vi "AFG3022_Arb_Fun_Control.vi"(10 "Channel":u16(ring) items=["Channel 1", "Channel 2"], 11 "Function Selector":u16(ring)=3 items=["Sine", "Square", "Ramp", "Assymetric Sine", "Assymetric Arbitrary"]) -> ()   [LabVIEW 2011]
panel:
  in  "Set Zero Mean":bool
  out "Amplitude":dbl
  in  "Set Amplitude":bool
  out "Ts/T":dbl=0.32
  in  "Time Ratio":dbl[](array[slide])=[0.07, 0.15, 0.1, 0.6799999999999999] min=0.0 max=1.0 step=0.01 scale=0.0..1.0
  in  "Fine Amp":dbl(knob) min=0.0 max=1.0 step=0.1 scale=0.0..1.0
  in  "Course Amp":dbl(knob)=1.0 min=-10.0 max=10.0 step=1.0 scale=-10.0..10.0
  in  "Channel 2":bool
  in  "Channel 1":bool=TRUE
  in  "Set Frequency":bool
  in  "Scale":u16(ring)=2 items=["1", "10", "100", "1k", "10k"]
  in  "Fine Freq":dbl(knob)=0.30000000000000004 min=0.0 max=1.0 step=0.1 scale=0.0..1.0
  in  "Course Freq":dbl(knob)=3.0 min=0.0 max=10.0 step=1.0 scale=0.0..10.0
  in  "Stop Button":bool
  in  "VISA resource name":refnum<visa-resource-name>="USB0::0x0699::0x0347::C036837::INSTR"
  out "Frequency":dbl=330.0
  # "Suction Time"
  # "Blowing Time"
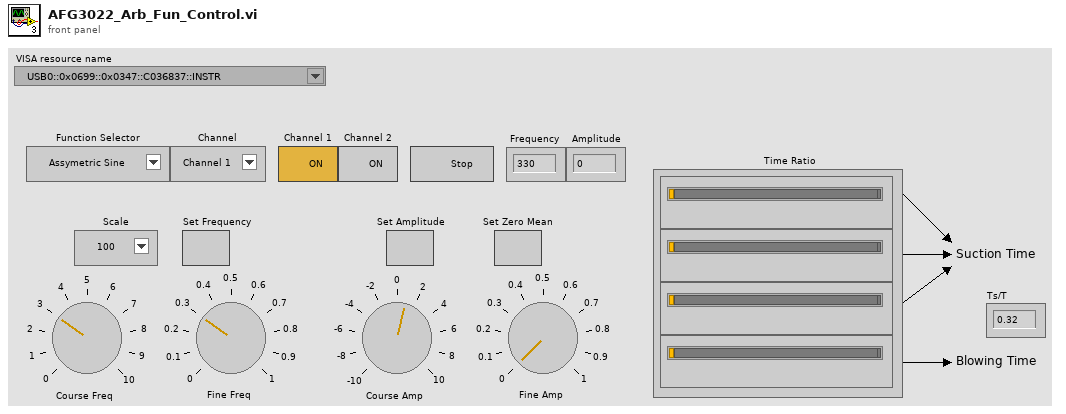
[diagram p1: front panel]
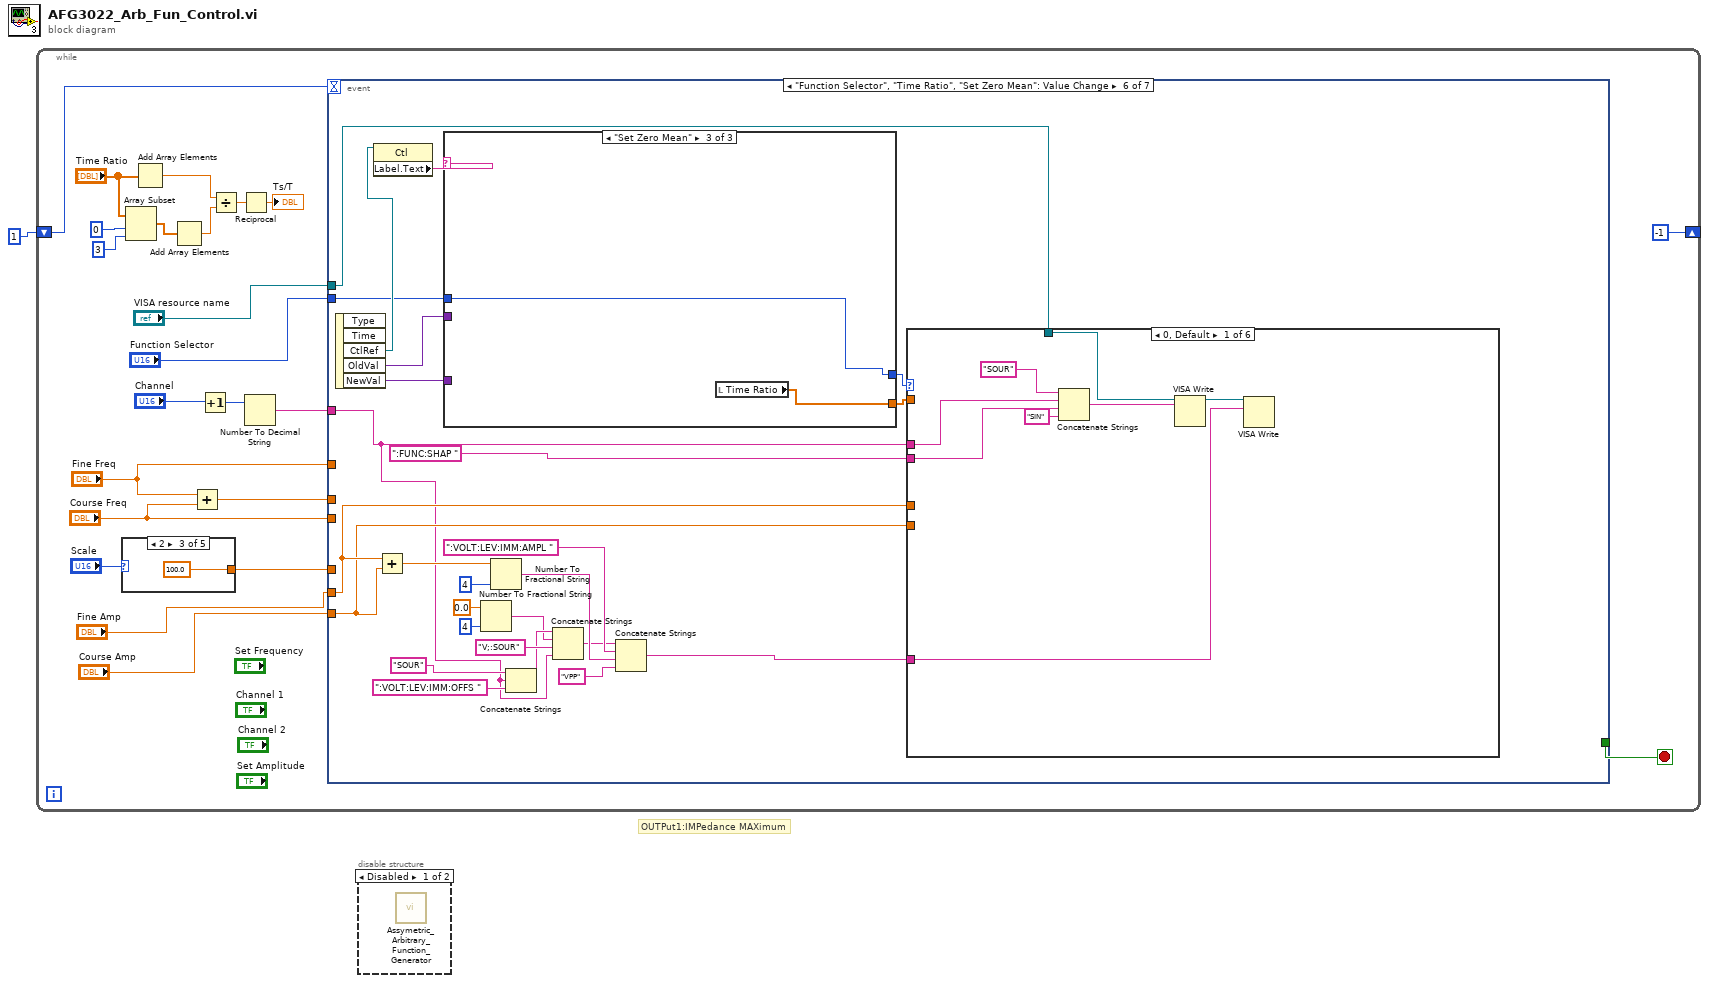
[diagram p0: block diagram]
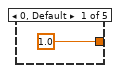
[diagram p3: hidden frame]
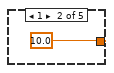
[diagram p4: hidden frame]
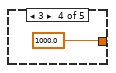
[diagram p5: hidden frame]
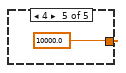
[diagram p6: hidden frame]
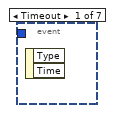
[diagram p7: hidden frame]
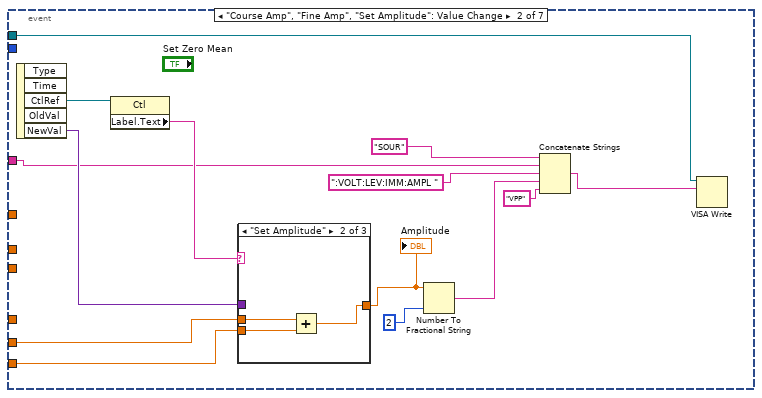
[diagram p8: hidden frame]
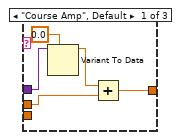
[diagram p9: hidden frame]
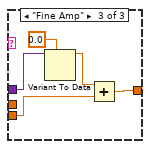
[diagram p10: hidden frame]
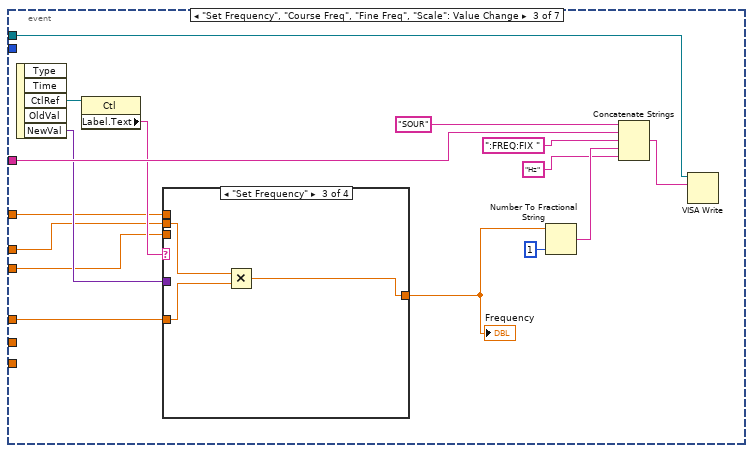
[diagram p11: hidden frame]
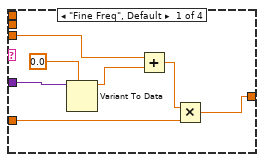
[diagram p12: hidden frame]
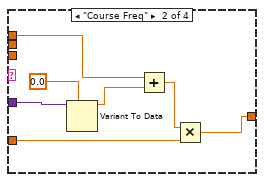
[diagram p13: hidden frame]
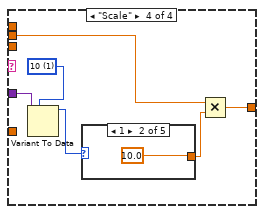
[diagram p14: hidden frame]
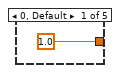
[diagram p15: hidden frame]
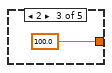
[diagram p16: hidden frame]
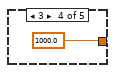
[diagram p17: hidden frame]
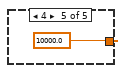
[diagram p18: hidden frame]
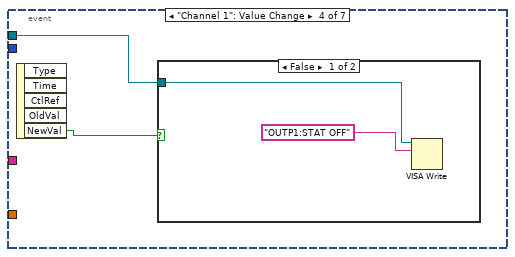
[diagram p19: hidden frame]
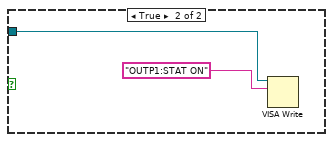
[diagram p20: hidden frame]
diagram:
  # "OUTPut1:IMPedance MAXimum"
  n1 = while {
    shift-right: [-1] -> _
    shift-left: 1 -> [w21]
    stop <- w23 stop-if-true
    n2 = case shown="2" "Scale" {
      tunnel: [1.0 10.0 100.0 1000.0 10000.0] -> w14
      frame 0, Default {
      }
      frame 1 {
      }
      frame 2 {
      }
      frame 3 {
      }
      frame 4 {
      }
    }
    n3 = Array Subset(array="Time Ratio", index=0, length=3) -> (w7:dbl[])
    n4 = Add Array Elements(numeric array="Time Ratio") -> (sum=w6:dbl)
    n5 = Add Array Elements(numeric array=w7) -> (sum=w5:dbl)
    n6 = Add(x="Fine Freq", y="Course Freq") -> (x+y=w16:dbl)
    n7 = Increment(x="Channel") -> (x+1=w19:u16)
    n8 = Divide(x=w6, y=w5) -> (x/y=w4:dbl)
    n9 = Reciprocal(x=w4) -> (1/x=→"Ts/T":dbl)
    n10 = Number To Decimal String(number=w19) -> (decimal integer string=w17:string)  [unwired: 1 in]
    n11 = event shown="[5] \"Function Selector\", \"Time Ratio\", \"Set Zero Mean\": Value Change" {
      selector: _ -> [_ _ _ _ _ _ _]
      dyn-events: _ -> [_ _ _ _ _ _ _]
      timeout: w21 -> [_ _ _ _ _ _ _]
      tunnel: "VISA resource name" -> [_ w30 w67 w102 w107 w138 _]
      tunnel: [_ _ _ _ _ _ "Stop Button"] -> w23
      tunnel: w17 -> [_ w31 w65 _ _ w116 _]
      tunnel: w16 -> [_ _ w61 _ _ _ _]
      tunnel: "Course Freq" -> [_ _ w59 _ _ _ _]
      tunnel: w14 -> [_ _ w58 _ _ _ _]
      tunnel: "Fine Freq" -> [_ _ w57 _ _ _ _]
      tunnel: "Course Amp" -> [_ w40 _ _ _ w118 _]
      tunnel: "Fine Amp" -> [_ w39 _ _ _ w119 _]
      tunnel: "Function Selector" -> [_ _ _ _ _ w114 _]
      event Timeout {
        n12 = event-data() -> ()  [unwired: 1 in, 2 out]
      }
      event "Course Amp", "Fine Amp", "Set Amplitude": Value Change {
        n13 = event-data() -> ("CtlRef"=w43:refnum<vi>, "NewVal"=w41:variant)  [unwired: 1 in, 3 out]
        n14 = property class="Ctl"(reference=w43) -> ("Label.Text"=w42:string)  [unwired: 1 in, 2 out]
        n15 = case shown="\"Set Amplitude\"" w42 {
          tunnel: w41 -> [w45 _ w53]
          tunnel: w40 -> [_ w50 w56]
          tunnel: w39 -> [w48 w51 _]
          tunnel: [w47 w49 w55] -> w38
          frame "Course Amp", Default {
            n16 = Variant To Data(type=0.0 ("Fine Amp"), Variant=w45) -> (data=w44:dbl)  [unwired: 1 in, 1 out]
            n17 = Add(x=w44, y=w48) -> (x+y=w47:dbl)
          }
          frame "Set Amplitude" {
            n18 = Add(x=w51, y=w50) -> (x+y=w49:dbl)
          }
          frame "Fine Amp" {
            n19 = Variant To Data(type=0.0 ("Fine Amp"), Variant=w53) -> (data=w52:dbl)  [unwired: 1 in, 1 out]
            n20 = Add(x=w52, y=w56) -> (x+y=w55:dbl)
          }
        }
        "Amplitude" <- w38
        n21 = Number To Fractional String(number=w38, precision (6)=i16 2) -> (F-format string=w33:string)  [unwired: 2 in]
        n22 = Concatenate Strings("SOUR" ("string"), w31, ":VOLT:LEV:IMM:AMPL " ("string"), w33, "VPP" ("string")) -> (w34:string)
        n23 = VISA Write(VISA resource name=w30, write buffer=w34) -> ()  [unwired: 1 in, 3 out]
      }
      event "Set Frequency", "Course Freq", "Fine Freq", "Scale": Value Change {
        n24 = event-data() -> ("CtlRef"=w64:refnum<vi>, "NewVal"=w62:variant)  [unwired: 1 in, 3 out]
        n25 = property class="Ctl"(reference=w64) -> ("Label.Text"=w63:string)  [unwired: 1 in, 2 out]
        n26 = case shown="\"Set Frequency\"" w63 {
          tunnel: w62 -> [w79 w86 _ w95]
          tunnel: w61 -> [_ _ w89 w91]
          tunnel: [w73 w80 w87 w90] -> w60
          tunnel: w59 -> [w76 _ _ _]
          tunnel: w58 -> [w74 w82 w88 _]
          tunnel: w57 -> [_ w81 _ _]
          frame "Fine Freq", Default {
            n27 = Variant To Data(type=0.0, Variant=w79) -> (data=w77:dbl)  [unwired: 1 in, 1 out]
            n28 = Add(x=w76, y=w77) -> (x+y=w75:dbl)
            n29 = Multiply(x=w75, y=w74) -> (x*y=w73:dbl)
          }
          frame "Course Freq" {
            n30 = Variant To Data(type=0.0, Variant=w86) -> (data=w84:dbl)  [unwired: 1 in, 1 out]
            n31 = Add(x=w81, y=w84) -> (x+y=w83:dbl)
            n32 = Multiply(x=w83, y=w82) -> (x*y=w80:dbl)
          }
          frame "Set Frequency" {
            n33 = Multiply(x=w89, y=w88) -> (x*y=w87:dbl)
          }
          frame "Scale" {
            w94 = u16 1 items=["1", "10", "100", "1k", "10k"] ("Scale")
            n34 = Variant To Data(type=w94, Variant=w95) -> (data=w93:u16)  [unwired: 1 in, 1 out]
            n35 = case shown="1" w93 {
              tunnel: [1.0 10.0 100.0 1000.0 10000.0] -> w92
              frame 0, Default {
              }
              frame 1 {
              }
              frame 2 {
              }
              frame 3 {
              }
              frame 4 {
              }
            }
            n36 = Multiply(x=w91, y=w92) -> (x*y=w90:dbl)
          }
        }
        "Frequency" <- w60
        n37 = Number To Fractional String(number=w60, precision (6)=i16 1) -> (F-format string=w69:string)  [unwired: 2 in]
        n38 = Concatenate Strings("SOUR", w65, ":FREQ:FIX " ("string"), w69, "Hz" ("string")) -> (w66:string)
        n39 = VISA Write(VISA resource name=w67, write buffer=w66) -> ()  [unwired: 1 in, 3 out]
      }
      event "Channel 1": Value Change {
        n40 = event-data() -> ("NewVal"=w101:bool)  [unwired: 1 in, 4 out]
        n41 = case shown="False" w101 {
          tunnel: w102 -> [w103 w106]
          frame False {
            n42 = VISA Write(VISA resource name=w103, write buffer="OUTP1:STAT OFF") -> ()  [unwired: 1 in, 3 out]
          }
          frame True {
            n43 = VISA Write(VISA resource name=w106, write buffer="OUTP1:STAT ON") -> ()  [unwired: 1 in, 3 out]
          }
        }
      }
      event "Channel 2": Value Change {
        n44 = event-data() -> ("NewVal"=w108:bool)  [unwired: 1 in, 4 out]
        n45 = case shown="False" w108 {
          tunnel: w107 -> [w109 w111]
          frame False {
            n46 = VISA Write(VISA resource name=w109, write buffer="OUTP2:STAT OFF") -> ()  [unwired: 1 in, 3 out]
          }
          frame True {
            n47 = VISA Write(VISA resource name=w111, write buffer="OUTP2:STAT ON") -> ()  [unwired: 1 in, 3 out]
          }
        }
      }
      event "Function Selector", "Time Ratio", "Set Zero Mean": Value Change {
        n48 = event-data() -> ("CtlRef"=w136:refnum<vi>, "OldVal"=w113:variant, "NewVal"=w134:variant)  [unwired: 1 in, 2 out]
        n49 = property class="Ctl"(reference=w136) -> ("Label.Text"=w135:string)  [unwired: 1 in, 2 out]
        n50 = Add(x=w119, y=w118) -> (x+y=w117:dbl)
        n51 = case shown="\"Set Zero Mean\"" w135 {
          tunnel: w134 -> [w146 w183 _]
          tunnel: [w145 w182 w185] -> w133
          tunnel: [w140 w181 w184] -> w132
          tunnel: w114 -> [w139 w180 w185]
          tunnel: w113 -> [w144 _ _]
          frame "Time Ratio" {
            w142 = dbl[] []
            n52 = Variant To Data(type=w142, Variant=w144) -> (data=w143:dbl[])  [unwired: 1 in, 1 out]
            n53 = Variant To Data(type=w142, Variant=w146) -> (data=w141:dbl[])  [unwired: 1 in, 1 out]
            n54 = case shown="3" w139 {
              selector: w139 -> [w147 w165]
              tunnel: [w147 w165] -> w145
              tunnel: w143 -> [w160 w179]
              tunnel: w141 -> [w151 w167]
              tunnel: [w148 w166] -> w140
              frame 4, Default {
                n55 = for {
                  tunnel: w160 -> [w164] mode=indexing
                  tunnel: w151 -> [w163] mode=indexing
                  tunnel: [w161] -> w159
                  i -> [w161]
                  stop <- w162 stop-if-true
                  n56 = Not Equal?(x=w164, y=w163) -> (x != y?=w162:bool)
                }
                n57 = Add Array Elements(numeric array=w151) -> (sum=w158:dbl)
                n58 = Decrement(x=w158) -> (x-1=w152:dbl)
                n59 = Equal?(x=3, y=w159) -> (x = y?=w156:bool)
                n60 = Select(t=1, s=w156, f=3 ("t")) -> (s? t:f=w149:i32)
                n61 = Index Array(array=w151, index=w149) -> (element=w153:dbl)
                n62 = Subtract(x=w153, y=w152) -> (x-y=w150:dbl)
                n63 = Replace Array Subset(array=w151, new element=w150, index=w149) -> (w148:dbl[])
                n64 = local write "Time Ratio"(w148) -> ()
              }
              frame 3 {
                w177 = 3 ("index")
                n65 = Index Array(array=w179, index=w177) -> (element=w178:dbl)
                n66 = Index Array(array=w167, index=w177) -> (element=w176:dbl)
                n67 = Not Equal?(x=w178, y=w176) -> (x != y?=w172:bool)
                n68 = Add Array Elements(numeric array=w167) -> (sum=w175:dbl)
                n69 = Decrement(x=w175) -> (x-1=w169:dbl)
                n70 = Select(t=1, s=w172, f=3 ("t")) -> (s? t:f=w171:i32)
                n71 = Index Array(array=w167, index=w171) -> (element=w170:dbl)
                n72 = Subtract(x=w170, y=w169) -> (x-y=w168:dbl)
                n73 = Replace Array Subset(array=w167, new element=w168, index=w171) -> (w166:dbl[])
                n74 = local write "Time Ratio"(w166) -> ()
              }
            }
          }
          frame "Function Selector", Default {
            n75 = Variant To Data(type=w180, Variant=w183) -> (data=w182:u16)  [unwired: 1 in, 1 out]
            n76 = local read "Time Ratio"() -> (w181:dbl[])
          }
          frame "Set Zero Mean" {
            n77 = local read "Time Ratio"() -> (w184:dbl[])
          }
        }
        n78 = Number To Fractional String(number=0.0, precision (6)=i16 4) -> (F-format string=w124:string)  [unwired: 2 in]
        n79 = Number To Fractional String(number=w117, precision (6)=i16 4) -> (F-format string=w129:string)  [unwired: 2 in]
        n80 = Concatenate Strings("SOUR" ("string"), w116, ":VOLT:LEV:IMM:OFFS " ("string")) -> (w125:string)
        n81 = Concatenate Strings(w125, w124, "V;:SOUR" ("string"), w116) -> (w127:string)
        n82 = Concatenate Strings(w127, ":VOLT:LEV:IMM:AMPL " ("string"), w129, "VPP" ("string")) -> (w115:string)
        n83 = case shown="0, Default" w133 {
          tunnel: w138 -> [w193 w198 w204 w233 w259 _]
          tunnel: w116 -> [w188 w197 w206 w220 w249 _]
          tunnel: ":FUNC:SHAP " ("string") -> [w191 w196 w205 _ _ _]
          tunnel: w119 -> [_ _ _ w236 w261 _]
          tunnel: w118 -> [_ _ _ w235 w260 _]
          tunnel: w132 -> [_ _ _ w214 w238 _]
          tunnel: w115 -> [w186 w195 w202 _ _ _]
          frame 0, Default {
            n84 = Concatenate Strings("SOUR" ("string"), w188, w191, "SIN" ("string")) -> (w189:string)
            n85 = VISA Write(VISA resource name=w193, write buffer=w189) -> (VISA resource name out=w187:refnum<visa-resource-name>)  [unwired: 1 in, 2 out]
            n86 = VISA Write(VISA resource name=w187, write buffer=w186) -> ()  [unwired: 1 in, 3 out]
          }
          frame 1 {
            n87 = Concatenate Strings("SOUR" ("string"), w197, w196, "SQU" ("string")) -> (w199:string)
            n88 = VISA Write(VISA resource name=w198, write buffer=w199) -> (VISA resource name out=w194:refnum<visa-resource-name>)  [unwired: 1 in, 2 out]
            n89 = VISA Write(VISA resource name=w194, write buffer=w195) -> ()  [unwired: 1 in, 3 out]
          }
          frame 2 {
            n90 = Concatenate Strings("SOUR" ("string"), w206, w205, "RAMP" ("string")) -> (w207:string)
            n91 = VISA Write(VISA resource name=w204, write buffer=w207) -> (VISA resource name out=w203:refnum<visa-resource-name>)  [unwired: 1 in, 2 out]
            n92 = VISA Write(VISA resource name=w203, write buffer=w202) -> ()  [unwired: 1 in, 3 out]
          }
          frame 3 {
            n93 = Add(x=w236, y=w235) -> (x+y=w234:dbl)
            n94 = Index Array(array=w214, index=3) -> (element=w213:dbl)
            n95 = Subtract(x=1.0, y=w213) -> (x-y=w211:dbl)
            n96 = Concatenate Strings("SOUR" ("string"), w220, ":VOLT:LEV:IMM:OFFS " ("string")) -> (w223:string)
            n97 = call "Assymetric_Sine_Wave.vi"("Ts"=w211, "Ub"=w234, "samples"=1000) -> ("offset"=w221:dbl, "amplitude"=w229:dbl, "Assymetric Sign Wave"=w232:dbl[])  [unwired: 6 in]
            n98 = Number To Fractional String(number=w221, precision (6)=i16 4) -> (F-format string=w224:string)  [unwired: 2 in]
            n99 = Number To Fractional String(number=w229, precision (6)=i16 4) -> (F-format string=w217:string)  [unwired: 2 in]
            n100 = call "Transfer_Arb_Waveform.vi"("Channel"=w220, "Arbitrary Waveform"=w232, "VISA resource name"=w233) -> ("error out"=w230:errorcluster, "VISA resource name out"=w231:refnum<visa-resource-name>)  [unwired: 7 in]
            n101 = Concatenate Strings(w223, w224, "V;:SOUR" ("string"), w220) -> (w219:string)
            n102 = Concatenate Strings(w219, ":VOLT:LEV:IMM:AMPL " ("string"), w217, "VPP" ("string")) -> (w215:string)
            n103 = VISA Write(VISA resource name=w231, write buffer=w215, error in (no error)=w230) -> ()  [unwired: 3 out]
          }
          frame 4 {
            n104 = Add(x=w261, y=w260) -> (x+y=w240:dbl)
            n105 = Concatenate Strings("SOUR" ("string"), w249, ":VOLT:LEV:IMM:OFFS " ("string")) -> (w251:string)
            n106 = call "Assymetric_Arbitrary_Wave.vi"("Time Ratios"=w238, "Ub"=w240, "samples"=1000) -> ("offset"=w241:dbl, "amplitude"=w242:dbl, "Arbitary Assymetric Waveform"=w243:dbl[])  [unwired: 6 in]
            n107 = Number To Fractional String(number=w241, precision (6)=i16 4) -> (F-format string=w252:string)  [unwired: 2 in]
            n108 = Number To Fractional String(number=w242, precision (6)=i16 4) -> (F-format string=w246:string)  [unwired: 2 in]
            n109 = call "Transfer_Arb_Waveform.vi"("Channel"=w249, "Arbitrary Waveform"=w243, "VISA resource name"=w259) -> ("error out"=w257:errorcluster, "VISA resource name out"=w258:refnum<visa-resource-name>)  [unwired: 7 in]
            n110 = Concatenate Strings(w251, w252, "V;:SOUR" ("string"), w249) -> (w248:string)
            n111 = Concatenate Strings(w248, ":VOLT:LEV:IMM:AMPL " ("string"), w246, "VPP" ("string")) -> (w244:string)
            n112 = VISA Write(VISA resource name=w258, write buffer=w244, error in (no error)=w257) -> ()  [unwired: 3 out]
          }
          frame 100 {
          }
        }
      }
      event "Stop Button": Value Change {
        n113 = event-data() -> ()  [unwired: 1 in, 5 out]
      }
    }
  }
  n114 = disable-structure shown="Disabled" {
    frame Disabled {
      n115 = call "Assymetric_Arbitrary_Function_Generator.vi"() -> ()  [unwired: 9 in, 3 out]
    }
    frame Enabled {
    }
  }
